vi "Goertz_end.vi"(2 "L_s(n-2)":dbl[](array[numeric]), 3 "L_s(n-1)":dbl[](array[numeric]), 4 "H_s(n-2)":dbl[](array[numeric]), 5 "H_s(n-1)":dbl[](array[numeric])) -> (0 "L_mag":dbl[](array[numeric]), 1 "H_mag":dbl[](array[numeric]))   [LabVIEW 2022 SP3]
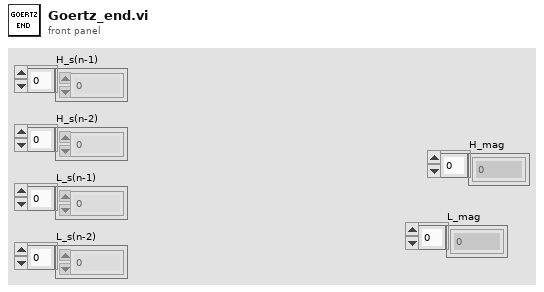
[diagram p1: front panel]
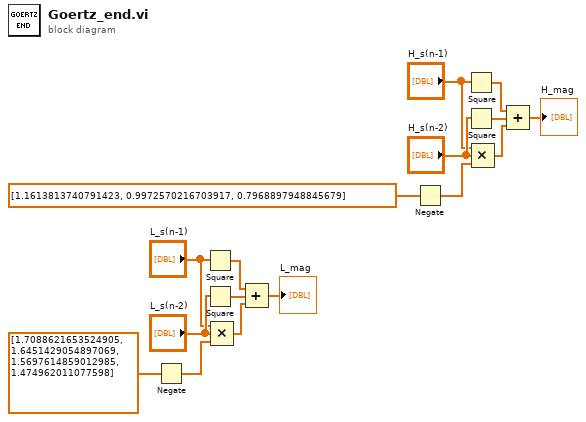
[diagram p0: block diagram]
diagram:
  n1 = Negate(x=dbl[] [1.7088621653524905, 1.6451429054897069, 1.5697614859012985, 1.474962011077598] ("2cos(L)")) -> (-x=w9:dbl[])
  n2 = Square(x="L_s(n-1)") -> (x^2=w10:dbl[])
  n3 = Square(x="L_s(n-2)") -> (x^2=w11:dbl[])
  n4 = Compound Arithmetic op=MULTIPLY("L_s(n-1)", "L_s(n-2)", w9) -> (w12:dbl[])
  n5 = Compound Arithmetic op=ADD(w10, w11, w12) -> (→"L_mag":dbl[])
  n6 = Negate(x=dbl[] [1.1613813740791423, 0.9972570216703917, 0.7968897948845679] ("2cos(H)")) -> (-x=w13:dbl[])
  n7 = Square(x="H_s(n-1)") -> (x^2=w3:dbl[])
  n8 = Square(x="H_s(n-2)") -> (x^2=w15:dbl[])
  n9 = Compound Arithmetic op=MULTIPLY("H_s(n-1)", "H_s(n-2)", w13) -> (w16:dbl[])
  n10 = Compound Arithmetic op=ADD(w3, w15, w16) -> (→"H_mag":dbl[])
